vi "CopyControls.vi"(0 "TemplateVIRef":refnum<vi>, 1 "TmplPanelRef":refnum<vi>, 2 "TmplControls[]":refnum<vi>[](array[refnum]), 3 "PanelRef":refnum<vi>, 4 "BlockDiagramRef":refnum<vi>, 5 "error in":errorcluster, 6 "CPref":refnum<vi>, 7 "TermUpper":i32, 8 "TmplWiringRules[]":T1(array[ring]), 9 "YSpacing":i32, 10 "ControlsToCopyIndex":i32[](array[numeric]), 11 "TermHorizontal":i32) -> (19 "error in":errorcluster)   [LabVIEW 2020, in "G#IDE.lvlib" / "ScriptingLib.lvlib"]
uses:
  ScriptingLib.lvlib
  <vilib>/Utility/miscctls.llb/LVPositionTypeDef.ctl
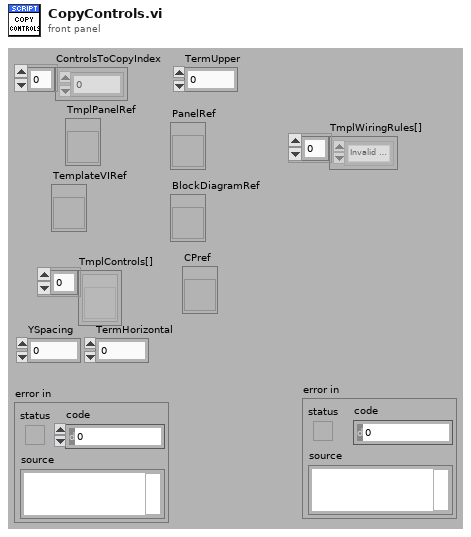
[diagram p1: front panel]
types:
  T1 = enum16{"Invalid Wire Rule", "Required", "Recommended", "Optional", "Dynamic Dispatch"}[]
  T2 = typedef "LVPositionTypeDef.ctl" = cluster{"Left":i32, "Top":i32}
  T3 = enum16{"Invalid Wire Rule", "Required", "Recommended", "Optional", "Dynamic Dispatch"}
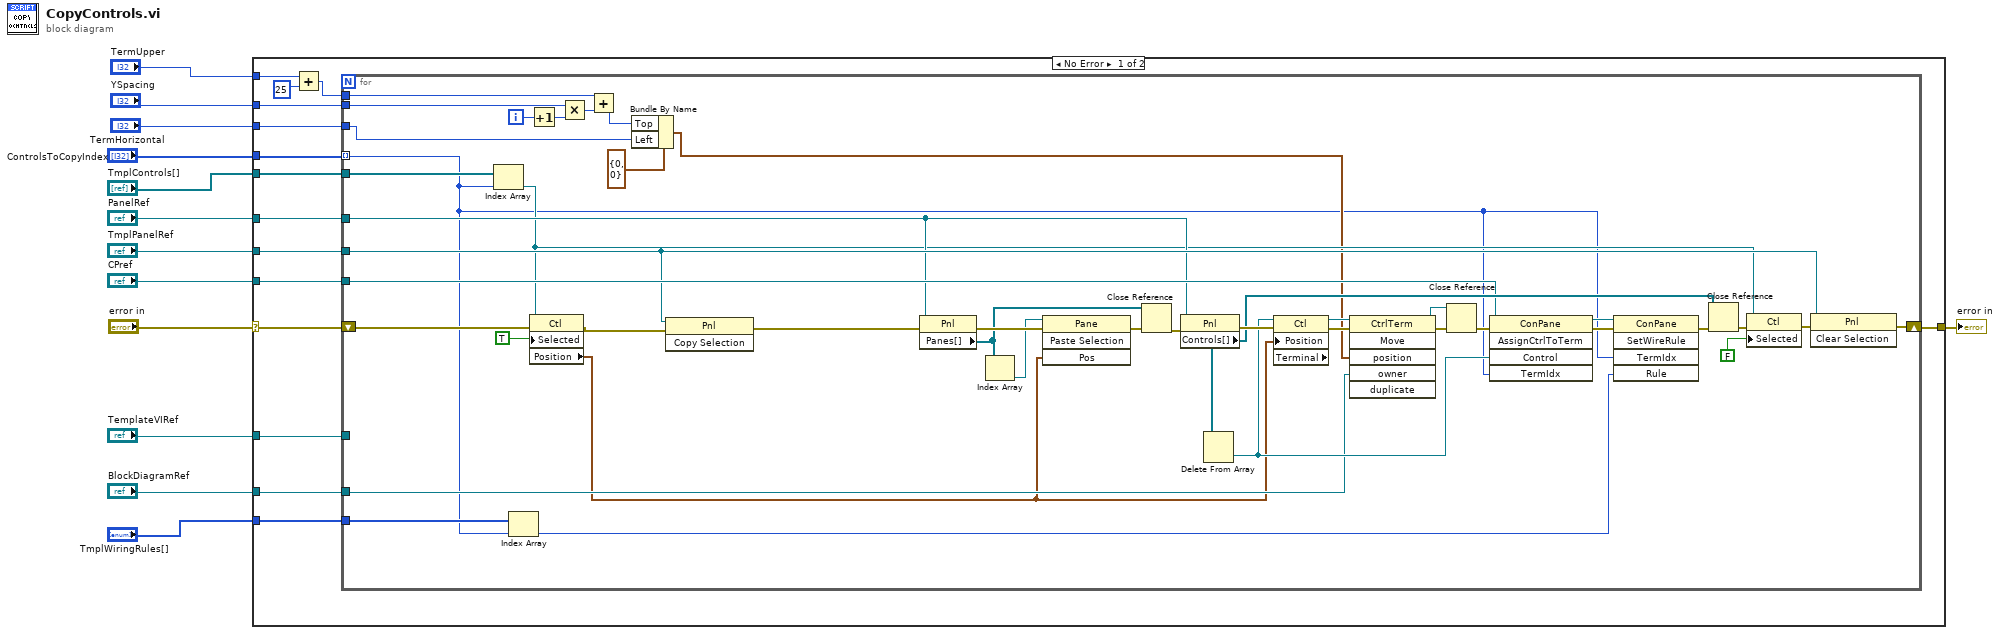
[diagram p0: block diagram]
diagram:
  n1 = case shown="No Error" "error in" {
    selector: "error in" -> [w19 w72]
    tunnel: "ControlsToCopyIndex" -> [w28 _]
    tunnel: "PanelRef" -> [w27 _]
    tunnel: "TmplPanelRef" -> [w26 _]
    tunnel: "CPref" -> [w25 _]
    tunnel: "TemplateVIRef" -> [w24 _]
    tunnel: "BlockDiagramRef" -> [w23 _]
    tunnel: "TmplWiringRules[]" -> [w22 _]
    tunnel: "TmplControls[]" -> [w21 _]
    tunnel: [w20 w72] -> w5
    tunnel: "TermUpper" -> [w16 _]
    tunnel: "YSpacing" -> [w18 _]
    tunnel: "TermHorizontal" -> [w17 _]
    frame No Error {
      n2 = Add(x=w16, y=25) -> (x+y=w15:i32)
      n3 = for {
        tunnel: w28 -> [w29] mode=indexing
        tunnel: w21 -> [w71]
        shift-right: [w54] -> w20
        shift-left: w19 -> [w69]
        tunnel: w26 -> [w44]
        tunnel: w27 -> [w43]
        tunnel: w25 -> [w45]
        tunnel: w22 -> [w62]
        tunnel: w23 -> [w41]
        tunnel: w24 -> [_]
        tunnel: w15 -> [w34]
        tunnel: w18 -> [w33]
        tunnel: w17 -> [w32]
        i -> [w36]
        n4 = Index Array(array=w71, index=w29) -> (element=w42:refnum<vi>)
        n5 = Index Array(array=w62, index=w29) -> (element=w61:T3)
        n6 = Increment(x=w36) -> (x+1=w35:i32)
        n7 = property class="Ctl"(reference=w42, error in=w69, "Selected"=TRUE) -> (error out=w30:errorcluster, "Position"=w40:T2)  [unwired: 1 out]
        n8 = Multiply(x=w33, y=w35) -> (x*y=w39:i32)
        n9 = Add(x=w34, y=w39) -> (x+y=w37:i32)
        n10 = Bundle By Name(cluster=T2 {"Left"=0, "Top"=0} ("Position"), "Top"=w37, "Left"=w32) -> (w31:T2)
        n11 = invoke class="Pnl" method="Copy Selection"(reference=w44, error in=w30) -> (error out=w53:errorcluster)  [unwired: 1 in, 2 out]
        n12 = property class="Pnl"(reference=w43, error in=w53) -> (error out=w52:errorcluster, "Panes[]"=w48:refnum<vi>[])  [unwired: 1 out]
        n13 = Index Array(array=w48) -> (element=w51:refnum<vi>)  [unwired: 1 in]
        n14 = invoke class="Pane" method="Paste Selection"(reference=w51, error in=w52, "Pos"=w40) -> (error out=w50:errorcluster)  [unwired: 1 in, 3 out]
        n15 = Close Reference(reference=w48, error in (no error)=w50) -> (error out=w49:errorcluster)
        n16 = property class="Pnl"(reference=w43, error in=w49) -> (error out=w66:errorcluster, "Controls[]"=w59:refnum<vi>[])  [unwired: 1 out]
        n17 = Delete From Array(array=w59) -> (deleted portion=w63:refnum<vi>)  [unwired: 2 in, 1 out]
        n18 = property class="Ctl"(reference=w63, error in=w66, "Position"=w40) -> (error out=w67:errorcluster, "Terminal"=w68:refnum<vi>)  [unwired: 1 out]
        n19 = invoke class="CtrlTerm" method="Move"(reference=w68, error in=w67, "position"=w31, "owner"=w41) -> (reference out=w46:refnum<vi>, error out=w47:errorcluster)  [unwired: 2 in, 4 out]
        n20 = Close Reference(reference=w46, error in (no error)=w47) -> (error out=w58:errorcluster)
        n21 = invoke class="ConPane" method="AssignCtrlToTerm"(reference=w45, error in=w58, "Control"=w63, "TermIdx"=w29) -> (reference out=w64:refnum<vi>, error out=w65:errorcluster)  [unwired: 1 in, 3 out]
        n22 = invoke class="ConPane" method="SetWireRule"(reference=w64, error in=w65, "TermIdx"=w29, "Rule"=w61) -> (error out=w60:errorcluster)  [unwired: 1 in, 4 out]
        n23 = Close Reference(reference=w59, error in (no error)=w60) -> (error out=w56:errorcluster)
        n24 = property class="Ctl"(reference=w42, error in=w56, "Selected"=FALSE) -> (error out=w55:errorcluster)  [unwired: 1 out]
        n25 = invoke class="Pnl" method="Clear Selection"(reference=w44, error in=w55) -> (error out=w54:errorcluster)  [unwired: 1 in, 2 out]
      }
    }
    frame Error {
    }
  }
  "error in" <- w5
